vi "Decimation Filtering for Single Block.vi"() -> ()   [LabVIEW 2023]
doc: "Demonstrates how to use the DFD Nyquist Design VI to design a decimation filter and use the DFD MRate Filtering for Single Block VI to process a single block of data with the decimation filter.\n\nComplete the following steps to use this VI.\n1) Run the VI.\n2) Set <B>Zero Phase?</B> to False, run this VI again, and observe the Signals graph.\n3) Use the zoom tool to observe the samples at the beginning of the Decimated Signal plot. \n4) Change the <B>Extension Type</B> option, run this VI again, and observe the Signals graph.\n5) Examine the block diagram to learn how to set the specifications."
uses:
  <vilib>/addons/Digital Filter Design/_Objects.llb/DFD Multirate Filtering Mode.ctl
  <vilib>/addons/Digital Filter Design/Multirate.llb/DFD MRate Filtering for Single Block (Wfm).vi
  <vilib>/addons/Digital Filter Design/NI_DigFilterLicensed.lvlib
  <vilib>/measure/NI_MABase.lvlib
panel:
  out "Signals":waveform(dbl)[](graph)=[{"t0"=timestamp(0 s since 1904-01-01), "dt"=1.0, "Y"=[]}, {"t0"=timestamp(0 s since 1904-01-01), "dt"=1.0, "Y"=[]}]
  in  "Extension Type":u16(ring) items=["Zero padding", "Symmetric", "Periodic"]
  in  "Zero Phase?":bool=TRUE
  # "Select Help>>Show Context Help and move the cursor over the VI icon for more information."
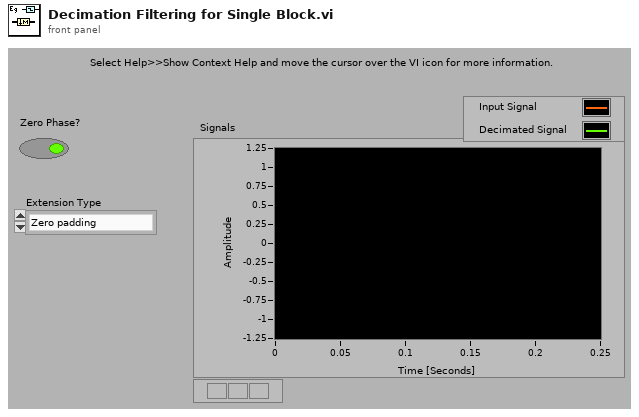
[diagram p1: front panel]
types:
  T1 = enum16{"Sine Wave", "Triangle Wave", "Square Wave", "Sawtooth Wave"}
  T2 = typedef "NI_DigFilterLicensed.lvlib/DFD Multirate Filtering Mode.ctl" = u16
  T3 = typedef "NI_DigFilterLicensed.lvlib/DFD Multirate Filter Obj.ctl" = cluster{"mMRate_Structure":enum16{"CIC", "FIR", "IIR", "Lattice"}, "mMRate_Mode":T4, "mMRate_Factor":i32, "mMRate_FIRParams":cluster{"mMRate_FIR_H":dbl[], "mMRate_FIR_IsNyquist?":bool, "mMRate_FIR_IsSymmetric?":bool}, "mMRate_CICParams":cluster{"mMRate_CIC_#Stage":i32, "mMRate_CIC_Lag":i32, "mMRate_CIC_Type":enum16{"Lowpass", "Highpass"}}, "mMRate_Order":i32, "mMRate_Version":string, "mMRate_Comments":string, "mMRate_RationalFactor":cluster{"mMRate_L":i32, "mMRate_M":i32}, "mMRate_Fs":dbl, "mMRate_Quantized?":bool, "mMRate_QFilterGain":dbl, "mMRate_CoefWl":i16, "mMRate_Scaling":cluster{"mMRate_ScaleByPowerOf2?":bool, "mMRate_ScaleType":T5}, "mMRate_InputWl":i16, "mMRate_OutputWl":i16, "mMRate_OutputMode":T6, "mMRate_MultMode":T7, "mMRate_BitPruning":bool, "mMRate_GainWl":i16, "mMRate_OutputFwl":i16, "mMRate_SumIwl":i16, "mMRate_InputIwl ":i16, "mMRate_SumWl":i16, "mMRate_CoefIwl":i16}
  T4 = typedef "NI_DigFilterLicensed.lvlib/DFD Multirate Mode.ctl" = i16
  T5 = typedef "NI_DigFilterLicensed.lvlib/DFD Coef Norm Type.ctl" = enum16{"No Norm", "Time Domain 1-Norm", "Time Domain 2-Norm", "Time Domain Inf-Norm"}
  T6 = typedef "NI_DigFilterLicensed.lvlib/DFD Round-off Mode.ctl" = enum16{"Nearest", "Truncation"}
  T7 = typedef "NI_DigFilterLicensed.lvlib/DFD FXP MRate Multiply Mode.ctl" = enum16{"Truncated", "Full"}
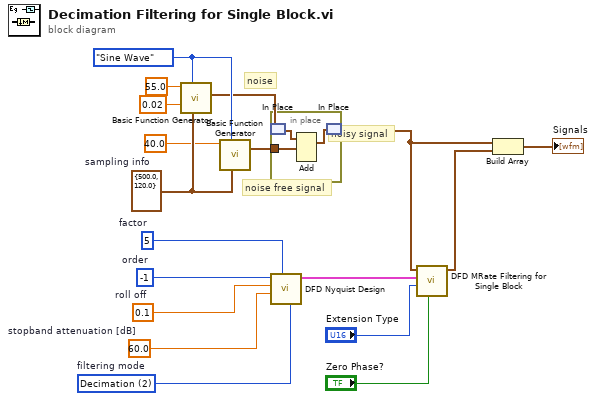
[diagram p0: block diagram]
diagram:
  w10 = T1."Sine Wave" ("signal type")
  w8 = cluster{"Fs":dbl, "#s":dbl} {"Fs"=500.0, "#s"=120.0}  # sampling info
  w11 = -1  # order
  w15 = 60.0  # stopband attenuation [dB]
  w16 = T2 2 items=["No Rate Change", "Interpolation", "Decimation"]  # filtering mode
  w17 = 0.1  # roll off
  w18 = 5  # factor
  # "noisy signal"
  # "noise free signal"
  # "noise"
  n1 = call <vilib>:"Basic Function Generator.vi"("sampling info"=w8, "signal type"=w10, "amplitude"=0.02, "frequency"=55.0) -> ("signal out"=w7:waveform(dbl))  [unwired: 5 in, 2 out]
  n2 = call <vilib>:"Basic Function Generator.vi"("sampling info"=w8, "signal type"=w10, "frequency"=40.0) -> ("signal out"=w9:waveform(dbl))  [unwired: 6 in, 2 out]
  n3 = in-place {
    in-place-border: w9 -> [w21]
    n4 = in-place-match #1(w7) -> (w20:waveform(dbl))
    n5 = Add(1:w21, 2:w20) -> (0:w19:waveform(dbl))  [unwired: 1 in, 1 out]
    n6 = in-place-match #1(w19) -> (w3:waveform(dbl))
  }
  n7 = call <vilib>:"DFD Nyquist Design.vi"("filtering mode"=w16, "factor"=w18, "stopband attenuation [dB]"=w15, "roll off"=w17, "order"=w11) -> ("multirate filter out"=w14:T3)  [unwired: 3 in, 3 out]
  n8 = call-poly <vilib>:"DFD MRate Filtering for Single Block.vi"("zero phase? (T)"="Zero Phase?", "extension type"="Extension Type", "multirate filter"=w14, "signal in"=w3) -> ("signal out"=w2:waveform(dbl))  [unwired: 1 in, 6 out]
  n9 = Build Array(w3, w2) -> (→"Signals":waveform(dbl)[])
